vi "get_elements_in_queue.vi"(11 "on-board buffer in":T1) -> (1 "empty?":bool, 2 "no. elements":u32)   [LabVIEW 2010, in "OnBoardBuffer.lvlib"]
uses:
  OnBoardBuffer.lvlib
  buffer_state_cluster.ctl
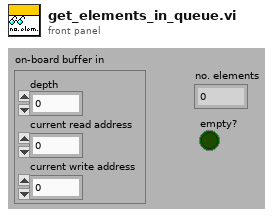
[diagram p1: front panel]
types:
  T1 = typedef "OnBoardBuffer.lvlib/buffer_state_cluster.ctl" = cluster{"depth":u32, "current read address":u32, "current write address":u32}
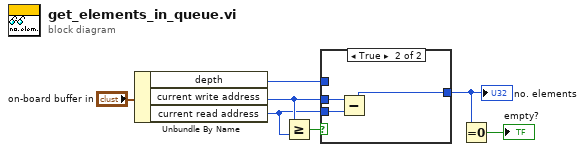
[diagram p0: block diagram]
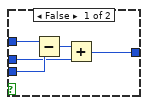
[diagram p2: hidden frame]
diagram:
  n1 = Unbundle By Name("on-board buffer in") -> ("depth"=w7:u32, "current write address"=w6:u32, "current read address"=w5:u32)
  n2 = Greater Or Equal?(x=w6, y=w5) -> (x >= y?=w4:bool)
  n3 = case shown="True" w4 {
    tunnel: w7 -> [w12 _]
    tunnel: w5 -> [w11 w15]
    tunnel: w6 -> [w9 w14]
    tunnel: [w8 w13] -> w2
    frame False {
      n4 = Subtract(x=w12, y=w11) -> (x-y=w10:u32)
      n5 = Add(x=w10, y=w9) -> (x+y=w8:u32)
    }
    frame True {
      n6 = Subtract(x=w14, y=w15) -> (x-y=w13:u32)
    }
  }
  "no. elements" <- w2
  n7 = Equal To 0?(x=w2) -> (x = 0?=→"empty?":bool)
